vi "UI_(01)_Set_startup_controls_state.vi"(3 "error in (no error)":errorcluster, 4 "Settings cluster in":T1={"Defaults"={"Default User"=0.0, "VISA Resource Name "=""}, "Recording and saving"={"Researcher name"="", "Name prefix"="", "Data post-processing"={"Filter type"=enum."Savitzky-Golay", "Length"=31, "Order"=3}, "Stop at"=0.0, "\"Stop at\" enabled"=FALSE, "Default save folder path"=path "", "Acquisition FPS"=enum."Max"}, "Geometry"={"Cage diameter, mm"=0, "Starting angle MIDFIELD"=0, "Starting angle BORDER"=0, "Radius, mm CENTER"=0, "Radius, mm MIDFIELD"=0, "N segments MIDFIELD"=0, "N segments BORDER"=0, "R-gap, mm"=0.0, "Bridge swap"=FALSE, "Bridge H. offset"=0.0, "Bridge V. offset"=0.0, "Twisted neck"=FALSE, "Alt. magn. orientation"=FALSE, "Sensor board size"=enum."Small"}, "IO parameters"={"IO general config."=0, "IO 1 configuration"=0, "IO 2 configuration"=0, "IO 3 configuration"=0, "IO 4 configuration"=0, "Activate ext. RS-232"=0, "IO inversion config."=0, "Sync capability"=1}, "Conditions presets array"=[{"Enabled"=FALSE, "Name"="", "Specifier(s)"=[], "Response"={"Response type"=enum."Air puff", "TTL port"=enum."Port 1", "TTL pulse length, ms"=0.0}, "Has been set"=FALSE}, {"Enabled"=FALSE, "Name"="", "Specifier(s)"=[], "Response"={"Response type"=enum."Air puff", "TTL port"=enum."Port 1", "TTL pulse length, ms"=0.0}, "Has been set"=FALSE}, {"Enabled"=FALSE, "Name"="", "Specifier(s)"=[], "Response"={"Response type"=enum."Air puff", "TTL port"=enum."Port 1", "TTL pulse length, ms"=0.0}, "Has been set"=FALSE}, {"Enabled"=FALSE, "Name"="", "Specifier(s)"=[], "Response"={"Response type"=enum."Air puff", "TTL port"=enum."Port 1", "TTL pulse length, ms"=0.0}, "Has been set"=FALSE}, {"Enabled"=FALSE, "Name"="", "Specifier(s)"=[], "Response"={"Response type"=enum."Air puff", "TTL port"=enum."Port 1", "TTL pulse length, ms"=0.0}, "Has been set"=FALSE}, {"Enabled"=FALSE, "Name"="", "Specifier(s)"=[], "Response"={"Response type"=enum."Air puff", "TTL port"=enum."Port 1", "TTL pulse length, ms"=0.0}, "Has been set"=FALSE}, {"Enabled"=FALSE, "Name"="", "Specifier(s)"=[], "Response"={"Response type"=enum."Air puff", "TTL port"=enum."Port 1", "TTL pulse length, ms"=0.0}, "Has been set"=FALSE}, {"Enabled"=FALSE, "Name"="", "Specifier(s)"=[], "Response"={"Response type"=enum."Air puff", "TTL port"=enum."Port 1", "TTL pulse length, ms"=0.0}, "Has been set"=FALSE}, {"Enabled"=FALSE, "Name"="", "Specifier(s)"=[], "Response"={"Response type"=enum."Air puff", "TTL port"=enum."Port 1", "TTL pulse length, ms"=0.0}, "Has been set"=FALSE}, {"Enabled"=FALSE, "Name"="", "Specifier(s)"=[], "Response"={"Response type"=enum."Air puff", "TTL port"=enum."Port 1", "TTL pulse length, ms"=0.0}, "Has been set"=FALSE}, {"Enabled"=FALSE, "Name"="", "Specifier(s)"=[], "Response"={"Response type"=enum."Air puff", "TTL port"=enum."Port 1", "TTL pulse length, ms"=0.0}, "Has been set"=FALSE}, {"Enabled"=FALSE, "Name"="", "Specifier(s)"=[], "Response"={"Response type"=enum."Air puff", "TTL port"=enum."Port 1", "TTL pulse length, ms"=0.0}, "Has been set"=FALSE}, {"Enabled"=FALSE, "Name"="", "Specifier(s)"=[], "Response"={"Response type"=enum."Air puff", "TTL port"=enum."Port 1", "TTL pulse length, ms"=0.0}, "Has been set"=FALSE}, {"Enabled"=FALSE, "Name"="", "Specifier(s)"=[], "Response"={"Response type"=enum."Air puff", "TTL port"=enum."Port 1", "TTL pulse length, ms"=0.0}, "Has been set"=FALSE}], "Calibration parameters"={"Timing calibration sw/hw"=1.0, "True FPS"=80.0, "True frame time, s"=80.0, "Disp. calibration info"=[]}, "Settings loaded OK"=FALSE} {"Calibration parameters"."True frame time, s" format="%.10g"; "Calibration parameters"."Disp. calibration info"."Speed, µl per ms" format="%.3g"; "Calibration parameters"."True FPS" format="%.10g"; "Calibration parameters"."Timing calibration sw/hw" format="%.10g"; "Conditions presets array"."Specifier(s)"."Validity criteria(s)"."Validity value" min=0.0 step=0.1 format="%.2g"; "Conditions presets array"."Specifier(s)"."Value" step=1.0 format="%#.2g"; "Recording and saving"."Data post-processing"."Order" min=3 max=11 step=2; "Recording and saving"."Data post-processing"."Length" min=5 max=301 step=2; "Geometry"."Cage diameter, mm" scale=0.0..340.0}, 5 "All references in":T18) -> (0 "error out":errorcluster, 1 "Settings cluster out":T1={"Defaults"={"Default User"=0.0, "VISA Resource Name "=""}, "Recording and saving"={"Researcher name"="", "Name prefix"="", "Data post-processing"={"Filter type"=enum."Savitzky-Golay", "Length"=31, "Order"=3}, "Stop at"=0.0, "\"Stop at\" enabled"=FALSE, "Default save folder path"=path "", "Acquisition FPS"=enum."Max"}, "Geometry"={"Cage diameter, mm"=0, "Starting angle MIDFIELD"=0, "Starting angle BORDER"=0, "Radius, mm CENTER"=0, "Radius, mm MIDFIELD"=0, "N segments MIDFIELD"=0, "N segments BORDER"=0, "R-gap, mm"=0.0, "Bridge swap"=FALSE, "Bridge H. offset"=0.0, "Bridge V. offset"=0.0, "Twisted neck"=FALSE, "Alt. magn. orientation"=FALSE, "Sensor board size"=enum."Small"}, "IO parameters"={"IO general config."=0, "IO 1 configuration"=0, "IO 2 configuration"=0, "IO 3 configuration"=0, "IO 4 configuration"=0, "Activate ext. RS-232"=0, "IO inversion config."=0, "Sync capability"=1}, "Conditions presets array"=[{"Enabled"=FALSE, "Name"="", "Specifier(s)"=[], "Response"={"Response type"=enum."Air puff", "TTL port"=enum."Port 1", "TTL pulse length, ms"=0.0}, "Has been set"=FALSE}, {"Enabled"=FALSE, "Name"="", "Specifier(s)"=[], "Response"={"Response type"=enum."Air puff", "TTL port"=enum."Port 1", "TTL pulse length, ms"=0.0}, "Has been set"=FALSE}, {"Enabled"=FALSE, "Name"="", "Specifier(s)"=[], "Response"={"Response type"=enum."Air puff", "TTL port"=enum."Port 1", "TTL pulse length, ms"=0.0}, "Has been set"=FALSE}, {"Enabled"=FALSE, "Name"="", "Specifier(s)"=[], "Response"={"Response type"=enum."Air puff", "TTL port"=enum."Port 1", "TTL pulse length, ms"=0.0}, "Has been set"=FALSE}, {"Enabled"=FALSE, "Name"="", "Specifier(s)"=[], "Response"={"Response type"=enum."Air puff", "TTL port"=enum."Port 1", "TTL pulse length, ms"=0.0}, "Has been set"=FALSE}, {"Enabled"=FALSE, "Name"="", "Specifier(s)"=[], "Response"={"Response type"=enum."Air puff", "TTL port"=enum."Port 1", "TTL pulse length, ms"=0.0}, "Has been set"=FALSE}, {"Enabled"=FALSE, "Name"="", "Specifier(s)"=[], "Response"={"Response type"=enum."Air puff", "TTL port"=enum."Port 1", "TTL pulse length, ms"=0.0}, "Has been set"=FALSE}, {"Enabled"=FALSE, "Name"="", "Specifier(s)"=[], "Response"={"Response type"=enum."Air puff", "TTL port"=enum."Port 1", "TTL pulse length, ms"=0.0}, "Has been set"=FALSE}, {"Enabled"=FALSE, "Name"="", "Specifier(s)"=[], "Response"={"Response type"=enum."Air puff", "TTL port"=enum."Port 1", "TTL pulse length, ms"=0.0}, "Has been set"=FALSE}, {"Enabled"=FALSE, "Name"="", "Specifier(s)"=[], "Response"={"Response type"=enum."Air puff", "TTL port"=enum."Port 1", "TTL pulse length, ms"=0.0}, "Has been set"=FALSE}, {"Enabled"=FALSE, "Name"="", "Specifier(s)"=[], "Response"={"Response type"=enum."Air puff", "TTL port"=enum."Port 1", "TTL pulse length, ms"=0.0}, "Has been set"=FALSE}, {"Enabled"=FALSE, "Name"="", "Specifier(s)"=[], "Response"={"Response type"=enum."Air puff", "TTL port"=enum."Port 1", "TTL pulse length, ms"=0.0}, "Has been set"=FALSE}, {"Enabled"=FALSE, "Name"="", "Specifier(s)"=[], "Response"={"Response type"=enum."Air puff", "TTL port"=enum."Port 1", "TTL pulse length, ms"=0.0}, "Has been set"=FALSE}, {"Enabled"=FALSE, "Name"="", "Specifier(s)"=[], "Response"={"Response type"=enum."Air puff", "TTL port"=enum."Port 1", "TTL pulse length, ms"=0.0}, "Has been set"=FALSE}], "Calibration parameters"={"Timing calibration sw/hw"=1.0, "True FPS"=80.0, "True frame time, s"=80.0, "Disp. calibration info"=[]}, "Settings loaded OK"=FALSE} {"Calibration parameters"."True frame time, s" format="%.10g"; "Calibration parameters"."Disp. calibration info"."Speed, µl per ms" format="%.3g"; "Calibration parameters"."True FPS" format="%.10g"; "Calibration parameters"."Timing calibration sw/hw" format="%.10g"; "Conditions presets array"."Specifier(s)"."Validity criteria(s)"."Validity value" min=0.0 step=0.1 format="%.2g"; "Conditions presets array"."Specifier(s)"."Value" step=1.0 format="%#.2g"; "Recording and saving"."Data post-processing"."Order" min=3 max=11 step=2; "Recording and saving"."Data post-processing"."Length" min=5 max=301 step=2; "Geometry"."Cage diameter, mm" scale=0.0..340.0}, 2 "All references out":T18)   [LabVIEW 2018, in "Tracker.lvlib"]
uses:
  Tracker.lvlib
  Controls/CTL_All_References.ctl
  Controls/CTL_Controls_References.ctl
  Controls/CTL_Indicators_References.ctl
  Controls/CTL_Panes_and_VIs_References.ctl
  Controls/CTL_Histogram_Properties.ctl
  <vilib>/Utility/miscctls.llb/LVRangeTypeDef.ctl
  Controls/CTL_Settings_cluster.ctl
  Controls/CTL_Filter_selector.ctl
  Controls/CTL_Acquisition_speed_selector.ctl
  Controls/CTL_Segmented_plot_parameters.ctl
  Controls/CTL_IO_params_cluster.ctl
  Controls/CTL_Conditions_Array.ctl
  Controls/CTL_Conditions_Cluster.ctl
  Controls/CTL_Condition_type.ctl
  Controls/CTL_Comparison_type.ctl
  Controls/CTL_Validity_check_criteria.ctl
  Controls/CTL_Response_info.ctl
  Controls/CTL_Condition_response_type.ctl
  Controls/CTL_Reponse_port_info.ctl
  Controls/CTL_Calibration_parameters.ctl
  Controls/CTL_Dispenser_calibration_info.ctl
  <vilib>/Utility/miscctls.llb/LVPointTypeDef.ctl
  <vilib>/Utility/error.llb/Error Cluster From Error Code.vi
  <vilib>/ErrorRing/Error Ring.xnode
panel:
  in  "Histogram initialization cluster":T16={"X Scale.Range"={"Minimum"=0.0, "Maximum"=13.0, "Increment"=1.0, "Minor Increment"=1.0, "Start"=0.0}, "Caption.Text"="Zone preference (normalized)", "X Scale.Offset and Multiplier:Multiplier"=1.0, "X Scale.Offset and Multiplier:Offset"=0.0, "X Scale.Scale Fit"=2, "X Scale.Display Format:Precision"=0, "Y Scale.Mapping Mode"=0, "Zones preference empty initialized array"=[0, 0, 0, 0, 0, 0, 0, 0, 0, 0, 0, 0, 0, 0], "Plot.Fill/Point Color"=15790320}
  out "Panes references":T21
  out "Controls references params":string[][](array[string])
  out "Indicators references params":string[][](array[string])
  out "Indicators references":T20
  out "Controls references":T19
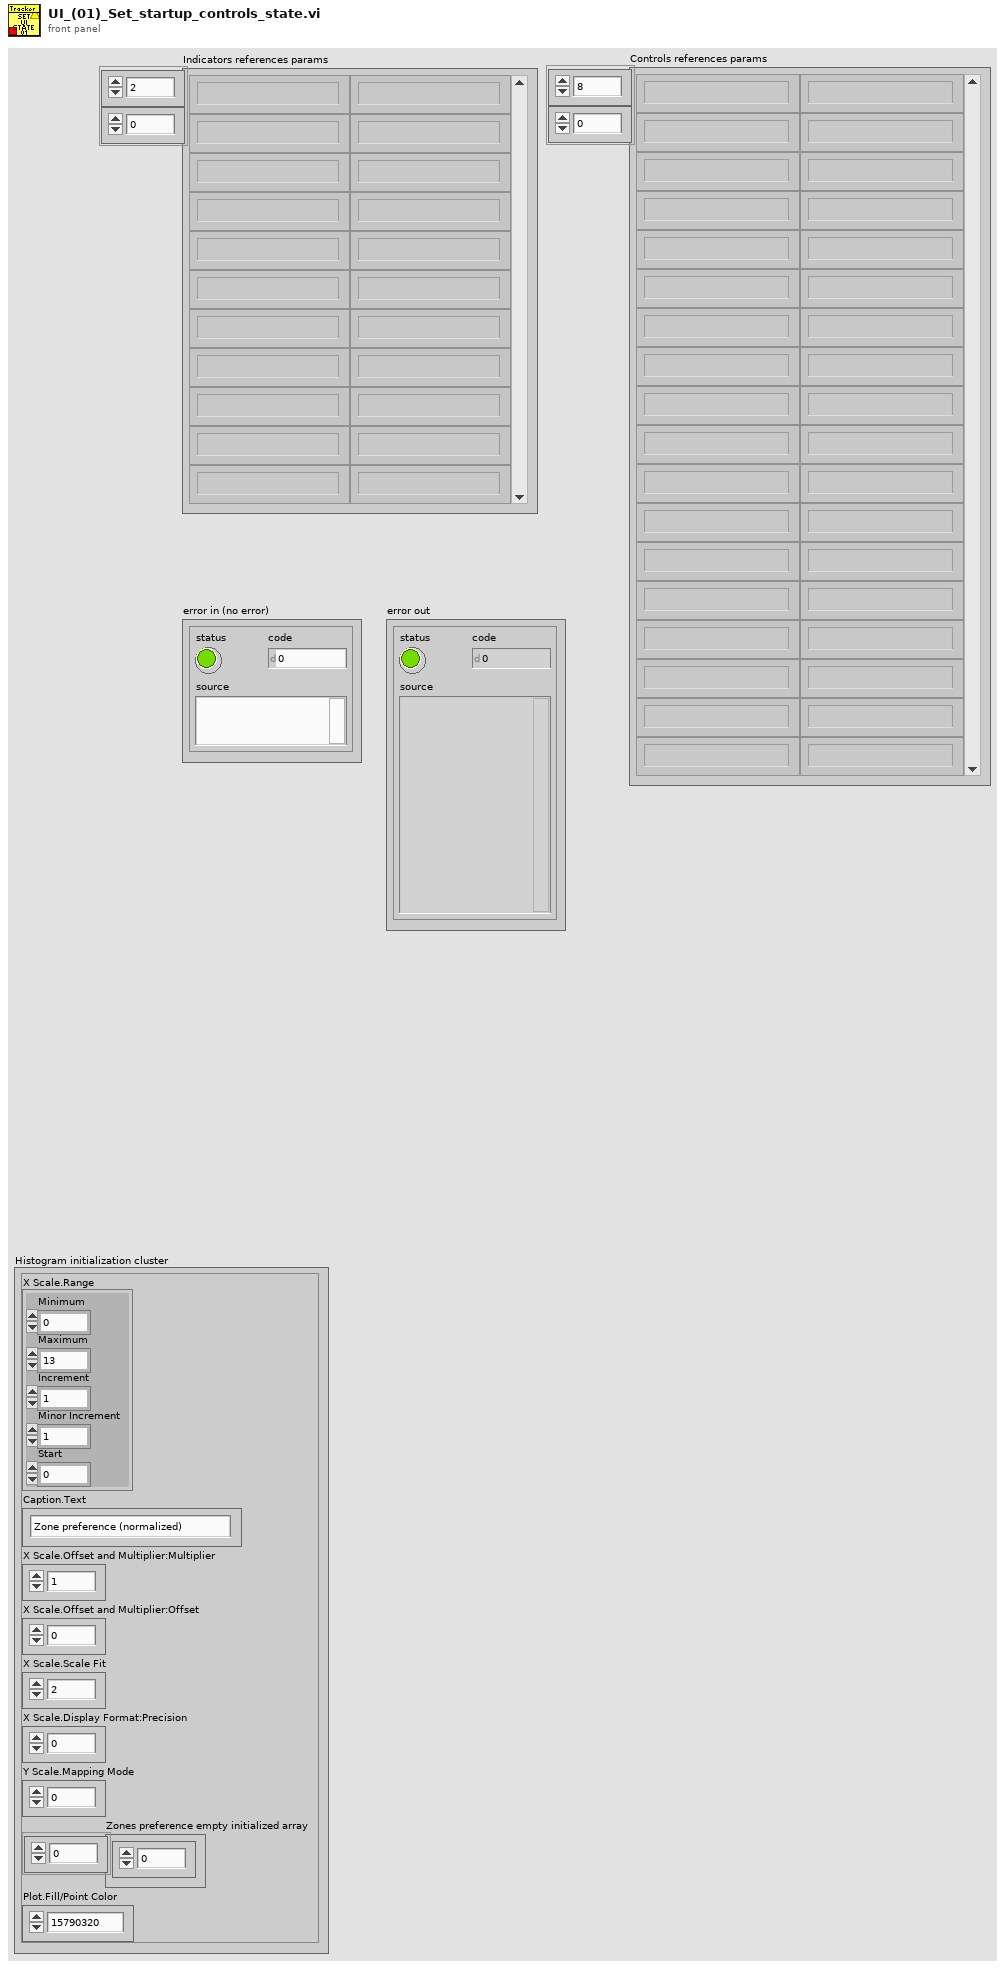
[diagram p1: front panel]
types:
  T1 = typedef "Tracker.lvlib/CTL_Settings_cluster.ctl" = cluster{"Defaults":cluster{"Default User":dbl, "VISA Resource Name ":string}, "Recording and saving":cluster{"Researcher name":string, "Name prefix":string, "Data post-processing":T2, "Stop at":dbl, "\"Stop at\" enabled":bool, "Default save folder path":path, "Acquisition FPS":T3}, "Geometry":T4, "IO parameters":T5, "Conditions presets array":T6, "Calibration parameters":T14, "Settings loaded OK":bool}
  T2 = typedef "Tracker.lvlib/CTL_Filter_selector.ctl" = cluster{"Filter type":enum16{"None", "Savitzky-Golay"}, "Length":i32, "Order":i32}
  T3 = typedef "Tracker.lvlib/CTL_Acquisition_speed_selector.ctl" = enum16{"Max", "Optimal", "Eco"}
  T4 = typedef "Tracker.lvlib/CTL_Segmented_plot_parameters.ctl" = cluster{"Cage diameter, mm":u16, "Starting angle MIDFIELD":i16, "Starting angle BORDER":i16, "Radius, mm CENTER":u16, "Radius, mm MIDFIELD":u16, "N segments MIDFIELD":u8, "N segments BORDER":u8, "R-gap, mm":sgl, "Bridge swap":bool, "Bridge H. offset":sgl, "Bridge V. offset":sgl, "Twisted neck":bool, "Alt. magn. orientation":bool, "Sensor board size":enum16{"Small", "Large"}}
  T5 = typedef "Tracker.lvlib/CTL_IO_params_cluster.ctl" = cluster{"IO general config.":u16, "IO 1 configuration":u16, "IO 2 configuration":u16, "IO 3 configuration":u16, "IO 4 configuration":u16, "Activate ext. RS-232":u16, "IO inversion config.":u16, "Sync capability":u8}
  T6 = typedef "Tracker.lvlib/CTL_Conditions_Array.ctl" = T7[]
  T7 = typedef "Tracker.lvlib/CTL_Conditions_Cluster.ctl" = cluster{"Enabled":bool, "Name":string, "Specifier(s)":cluster{"Specifier enabled":bool, "Condition type":T8, "Comparison type":T9, "Value":dbl, "Validity criteria(s)":cluster{"V. check enabled":bool, "Criteria":T10, "Validity value":dbl}[]}[], "Response":T11, "Has been set":bool}
  T8 = typedef "Tracker.lvlib/CTL_Condition_type.ctl" = enum16{"Speed", "Zone", "Angle to wall"}
  T9 = typedef "Tracker.lvlib/CTL_Comparison_type.ctl" = enum16{"Less", "Less or Equal", "Equal", "Greater or Equal", "Greater", "Not Equal"}
  T10 = typedef "Tracker.lvlib/CTL_Validity_check_criteria.ctl" = enum16{"Running bout (seconds)", "Running bout (meters)"}
  T11 = typedef "Tracker.lvlib/CTL_Response_info.ctl" = cluster{"Response type":T12, "TTL port":T13, "TTL pulse length, ms":dbl}
  T12 = typedef "Tracker.lvlib/CTL_Condition_response_type.ctl" = enum16{"None", "Air puff", "Liquid reward"}
  T13 = typedef "Tracker.lvlib/CTL_Reponse_port_info.ctl" = enum16{"Port 1", "Port 2", "Port 3", "Port 4"}
  T14 = typedef "Tracker.lvlib/CTL_Calibration_parameters.ctl" = cluster{"Timing calibration sw/hw":dbl, "True FPS":dbl, "True frame time, s":dbl, "Disp. calibration info":T15}
  T15 = typedef "Tracker.lvlib/CTL_Dispenser_calibration_info.ctl" = cluster{"Channel":u8, "Speed, µl per ms":dbl}[]
  T16 = typedef "Tracker.lvlib/CTL_Histogram_Properties.ctl" = cluster{"X Scale.Range":T17, "Caption.Text":string, "X Scale.Offset and Multiplier:Multiplier":dbl, "X Scale.Offset and Multiplier:Offset":dbl, "X Scale.Scale Fit":u8, "X Scale.Display Format:Precision":u8, "Y Scale.Mapping Mode":u8, "Zones preference empty initialized array":i32[], "Plot.Fill/Point Color":u32}
  T17 = typedef "LVRangeTypeDef.ctl" = cluster{"Minimum":dbl, "Maximum":dbl, "Increment":dbl, "Minor Increment":dbl, "Start":dbl}
  T18 = typedef "Tracker.lvlib/CTL_All_References.ctl" = cluster{"Controls references":T19, "Indicators references":T20, "Service references":T21}
  T19 = typedef "Tracker.lvlib/CTL_Controls_References.ctl" = cluster{"Check HW connection":refnum<vi>, "Save settings":refnum<vi>, "Reset zones":refnum<vi>, "Reset stimuli":refnum<vi>, "Record/Stop":refnum<vi>, "Reset barplot":refnum<vi>, "Multiplyer of chart RX":refnum<vi>, "Show zones":refnum<vi>, "Show magnets":refnum<vi>, "Show heatmap":refnum<vi>, "Show full track":refnum<vi>, "Open File":refnum<vi>, "Play/Pause":refnum<vi>, "Trace, s":refnum<vi>, "Playback speed":refnum<vi>, "Timeline":refnum<vi>, "By Zone stim. setup":refnum<vi>, "Set/Rec and Analyse Tab":refnum<vi>, "Cage radial segmentation":refnum<vi>, "Set IO config":refnum<vi>, "Rainbow (time)":refnum<vi>, "Rainbow (speed)":refnum<vi>, "Add Reward":refnum<vi>, "Modify Reward":refnum<vi>, "Delete Reward":refnum<vi>}
  T20 = typedef "Tracker.lvlib/CTL_Indicators_References.ctl" = cluster{"HW info":refnum<vi>, "Port":refnum<vi>, "Ready":refnum<vi>, "IO status indicator":refnum<vi>, "Current Time":refnum<vi>, "Record timestamp":refnum<vi>, "Mouse speed":refnum<vi>, "Mouse speed, mm/s":refnum<vi>, "Running, perc. of time":refnum<vi>, "Histograms":refnum<vi>, "Cage size":refnum<vi>, "Reward":refnum<vi>, "Current zone":refnum<vi>}
  T21 = typedef "Tracker.lvlib/CTL_Panes_and_VIs_References.ctl" = cluster{"Pane":refnum<vi>, "This VI":refnum<vi>, "Menu":refnum<k9>}
  T22 = typedef "LVPointTypeDef.ctl" = cluster{"Horizontal":i16, "Vertical":i16}
  T23 = enum8{"Enabled", "Disabled", "Disabled and Grayed Out"}
  T24 = enum32{"Page Enabled", "Page Disabled", "Page Disabled & Grayed"}
  T25 = cluster{"Slider":dbl, "Slider":dbl, "Slider":dbl}
  T26 = typedef "Tracker.lvlib/CTL_IO_status_indicator.ctl" = cluster{"IO1":bool, "IO2":bool, "IO3":bool, "IO4":bool, "St1":bool, "St2":bool, "St3":bool, "St4":bool, "Z1":bool, "Z2":bool, "Z3":bool, "Z4":bool, "Syn1":bool, "Syn2":bool, "RS-232 ext. activated":bool}
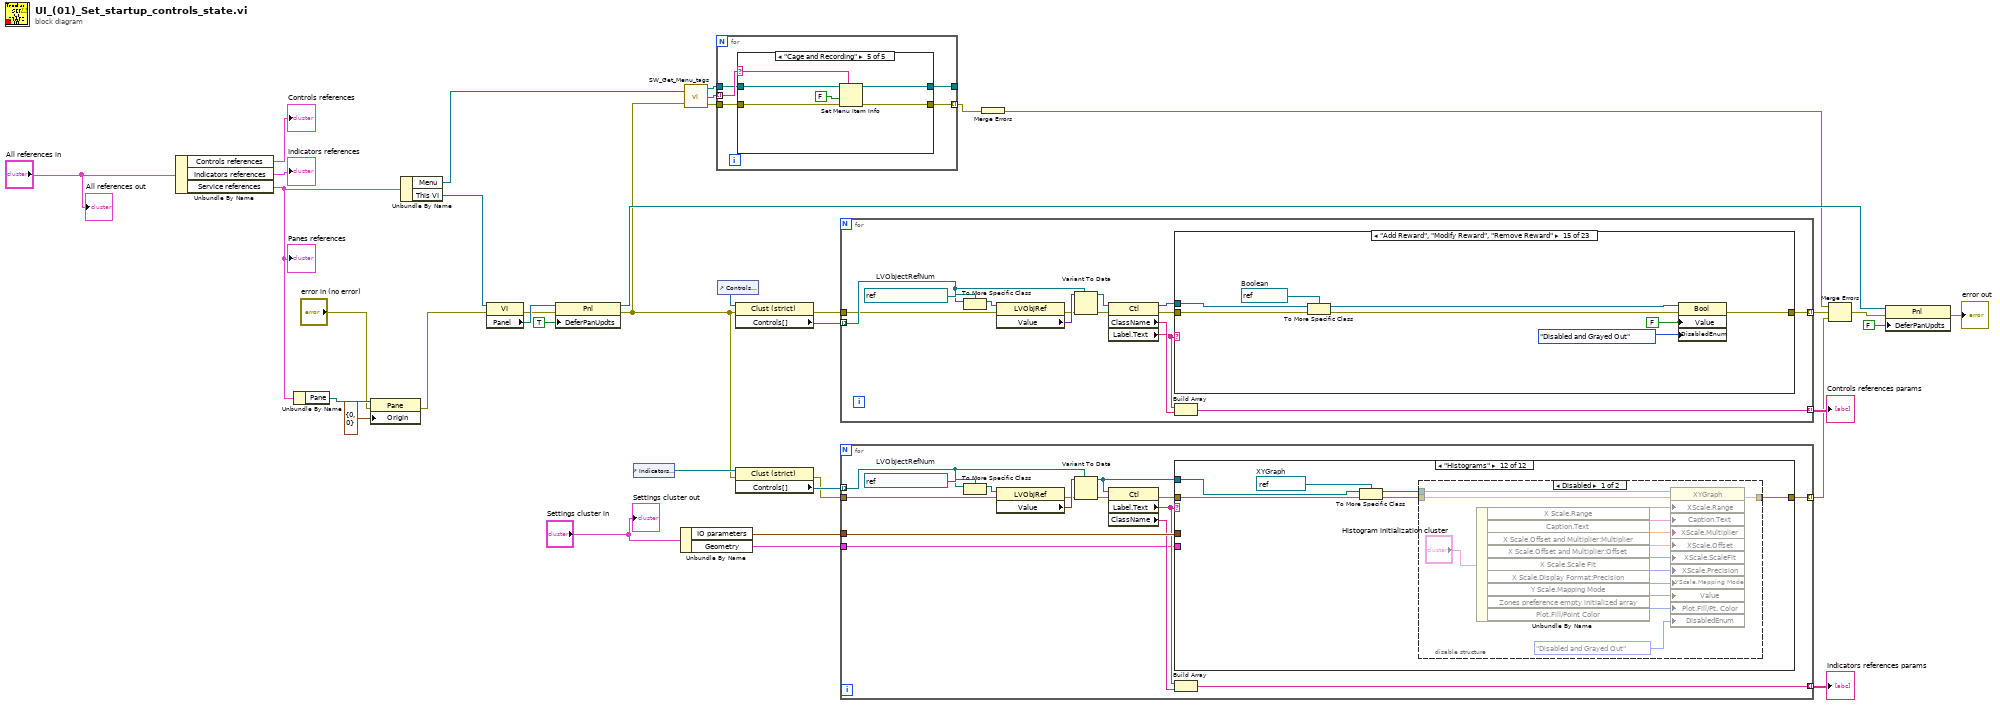
[diagram p0: block diagram]
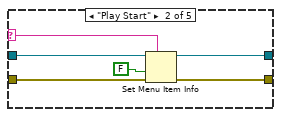
[diagram p3: hidden frame]
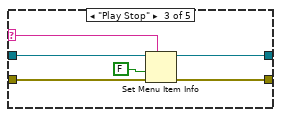
[diagram p4: hidden frame]
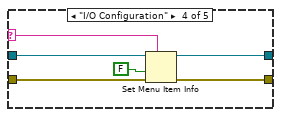
[diagram p5: hidden frame]
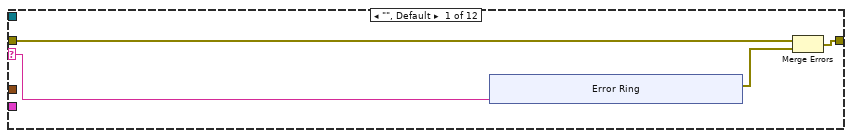
[diagram p6: hidden frame]
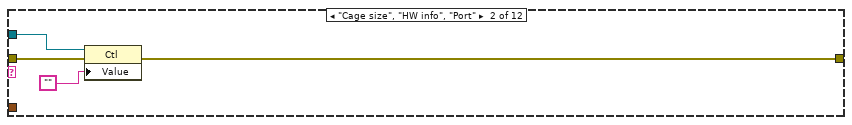
[diagram p7: hidden frame]
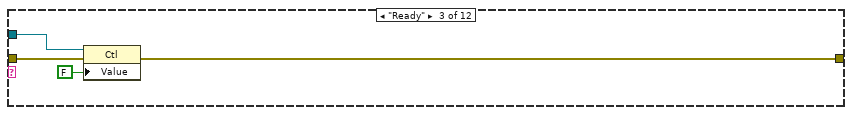
[diagram p8: hidden frame]
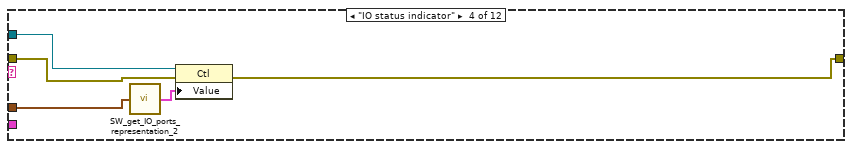
[diagram p9: hidden frame]
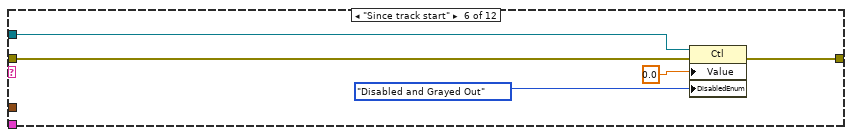
[diagram p11: hidden frame]
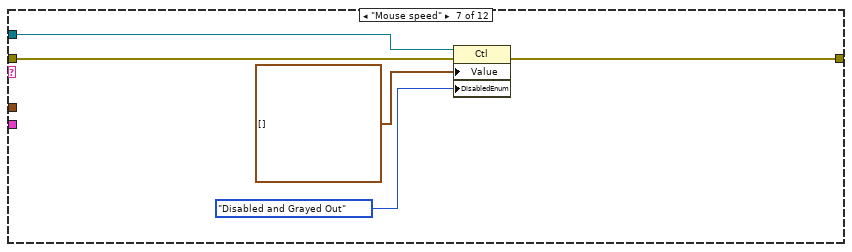
[diagram p12: hidden frame]
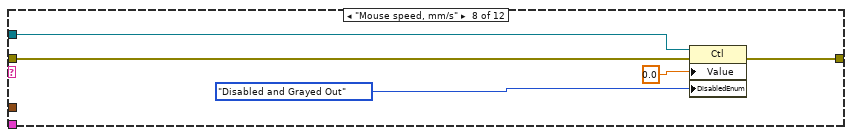
[diagram p13: hidden frame]
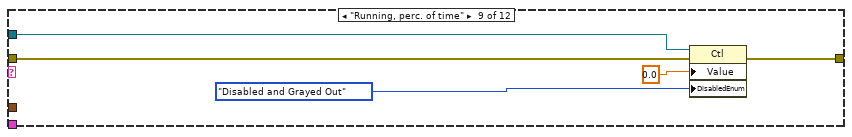
[diagram p14: hidden frame]
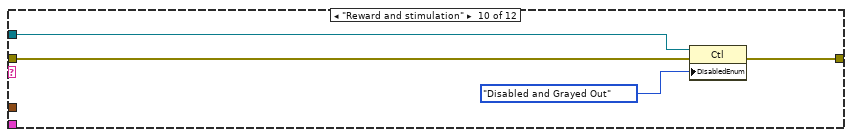
[diagram p15: hidden frame]
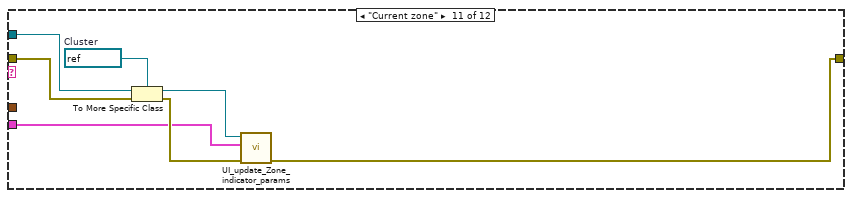
[diagram p16: hidden frame]
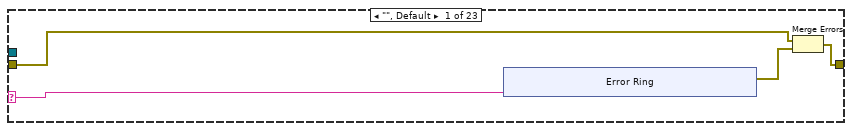
[diagram p18: hidden frame]
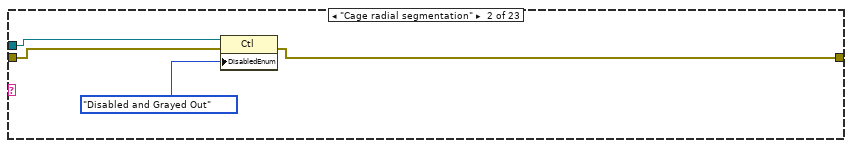
[diagram p19: hidden frame]
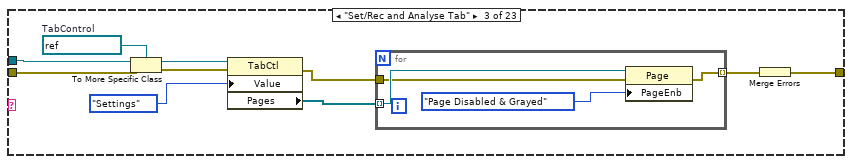
[diagram p20: hidden frame]
diagram:
  n1 = Unbundle By Name("All references in") -> ("Controls references"=→"Controls references":T19, "Indicators references"=→"Indicators references":T20, "Service references"=w14:T21)
  "Panes references" <- w14
  n2 = Unbundle By Name(w14) -> ("Pane"=w13:refnum<vi>)
  n3 = property class="Pane"(reference=w13, error in="error in (no error)", "Origin"=T22 {"Horizontal"=0, "Vertical"=0}) -> (error out=w11:errorcluster)  [unwired: 1 out]
  n4 = Unbundle By Name(w14) -> ("Menu"=w9:refnum<k9>, "This VI"=w25:refnum<vi>)
  n5 = property class="VI"(reference=w25, error in=w11) -> (error out=w18:errorcluster, "Panel"=w27:refnum<vi>)  [unwired: 1 out]
  n6 = property class="Pnl"(reference=w27, error in=w18, "DeferPanUpdts"=TRUE ("Defer Panel Updates")) -> (reference out=w19:refnum<vi>, error out=w8:errorcluster)
  n7 = control-ref of="Indicators references"() -> (w30:refnum<vi>)
  n8 = Unbundle By Name("Settings cluster in") -> ("IO parameters"=w15:T5, "Geometry"=w1:T4)
  n9 = call "SW_Get_Menu_tags.vi"("Menu ref in"=w9, "error in (no error)"=w8) -> ("Menu ref out"=w5:refnum<k9>, "(Sub)menu tags"=w7:string[], "error out"=w6:errorcluster)
  n10 = for {
    tunnel: w7 -> [w41] mode=indexing
    tunnel: w6 -> [w40]
    tunnel: [w39] -> w4 mode=indexing
    tunnel: [w38] -> _
    tunnel: w5 -> [w37]
    n11 = case shown="\"Cage and Recording\"" w41 {
      selector: w41 -> [_ w49 w55 w61 w67]
      tunnel: w40 -> [w43 w47 w53 w59 w65]
      tunnel: [w43 w46 w52 w58 w64] -> w39
      tunnel: [w42 w45 w51 w57 w63] -> w38
      tunnel: w37 -> [w42 w44 w50 w56 w62]
      frame "", Default {
      }
      frame "Play Start" {
        n12 = Set Menu Item Info(7:w49, 8:w47, 9:FALSE ("enabled"), 11:w44) -> (0:w46:errorcluster, 3:w45:refnum<k9>)  [unwired: 3 in]
      }
      frame "Play Stop" {
        n13 = Set Menu Item Info(7:w55, 8:w53, 9:FALSE ("enabled"), 11:w50) -> (0:w52:errorcluster, 3:w51:refnum<k9>)  [unwired: 3 in]
      }
      frame "I/O Configuration" {
        n14 = Set Menu Item Info(7:w61, 8:w59, 9:FALSE ("enabled"), 11:w56) -> (0:w58:errorcluster, 3:w57:refnum<k9>)  [unwired: 3 in]
      }
      frame "Cage and Recording" {
        n15 = Set Menu Item Info(7:w67, 8:w65, 9:FALSE ("enabled"), 11:w62) -> (0:w64:errorcluster, 3:w63:refnum<k9>)  [unwired: 3 in]
      }
    }
  }
  n16 = control-ref of="Controls references"() -> (w32:refnum<vi>)
  n17 = property class="Clust (strict)"(reference=w32, error in=w8) -> (error out=w24:errorcluster, "Controls[]"=w33:refnum<vi>[])  [unwired: 1 out]
  n18 = property class="Clust (strict)"(reference=w30, error in=w8) -> (error out=w23:errorcluster, "Controls[]"=w31:refnum<vi>[])  [unwired: 1 out]
  n19 = for {
    tunnel: w33 -> [w78] mode=indexing
    tunnel: [w75] -> w28 mode=indexing
    tunnel: w24 -> [w74]
    tunnel: [w70] -> w16 mode=indexing
    w80 = refnum<vi> refnum  # LVObjectRefNum
    n20 = To More Specific Class(target class=w80, reference=w78) -> (specific class reference=w81:refnum<vi>)  [unwired: 1 in, 1 out]
    n21 = property class="LVObjRef"(reference=w81, error in=w74) -> (error out=w73:errorcluster, "Value"=w79:variant)  [unwired: 1 out]
    n22 = Variant To Data(error in=w73, type=w78, Variant=w79) -> (data=w77:refnum<vi>, error out=w72:errorcluster)
    n23 = property class="Ctl"(reference=w77, error in=w72) -> (reference out=w68:refnum<vi>, error out=w69:errorcluster, "ClassName"=w76:string, "Label.Text"=w71:string)
    n24 = case shown="\"Add Reward\", \"Modify Reward\", \"Remove Reward\"" w71 {
      selector: w71 -> [w82 _ _ _ _ _ _ _ _ _ _ _ _ _ _ _ _ _ _ _ _ _ _]
      tunnel: [w84 w93 w97 w113 w121 w129 w137 w145 w153 w161 w169 w177 w185 w193 w201 w209 w217 w225 w233 w241 w249 w264 w271] -> w70
      tunnel: w69 -> [w85 w94 w101 w115 w123 w131 w139 w147 w155 w163 w171 w179 w187 w195 w203 w211 w219 w227 w235 w243 w251 w266 w273]
      tunnel: w68 -> [_ w96 w106 w118 w126 w134 w142 w150 w158 w166 w174 w182 w190 w198 w206 w214 w222 w230 w238 w246 w254 w269 w276]
      frame "", Default {
        n25 = xnode "Error Ring"("parameter 0"=w82) -> ("error out"=w83:errorcluster)
        n26 = Merge Errors(w85, w83) -> (w84:errorcluster)
      }
      frame "Cage radial segmentation" {
        n27 = property class="Ctl"(reference=w96, error in=w94, "DisabledEnum"=T23."Disabled and Grayed Out" ("Disabled")) -> (error out=w93:errorcluster)  [unwired: 1 out]
      }
      frame "Set/Rec and Analyse Tab" {
        w103 = refnum<vi> refnum  # TabControl
        n28 = To More Specific Class(target class=w103, reference=w106, error in=w101) -> (specific class reference=w104:refnum<vi>, error out=w100:errorcluster)
        n29 = property class="TabCtl"(reference=w104, error in=w100, "Value"=enum32{"Settings", "Recording and Analysis"}."Settings") -> (error out=w99:errorcluster, "Pages"=w102:refnum<vi>[])  [unwired: 1 out]
        n30 = for {
          tunnel: w102 -> [w109] mode=indexing
          tunnel: w99 -> [w108]
          tunnel: [w107] -> w98 mode=indexing
          n31 = property class="Page"(reference=w109, error in=w108, "PageEnb"=T24."Page Disabled & Grayed" ("Page Enabled State")) -> (error out=w107:errorcluster)  [unwired: 1 out]
        }
        n32 = Merge Errors(w98) -> (w97:errorcluster)
      }
      frame "Check HW connection" {
        w117 = refnum<vi> refnum  # Boolean
        n33 = To More Specific Class(target class=w117, reference=w118, error in=w115) -> (specific class reference=w116:refnum<vi>, error out=w114:errorcluster)
        n34 = property class="Bool"(reference=w116, error in=w114, "Value"=FALSE, "DisabledEnum"=T23."Disabled and Grayed Out" ("Disabled")) -> (error out=w113:errorcluster)  [unwired: 1 out]
      }
      frame "Save settings" {
        w125 = refnum<vi> refnum  # Boolean
        n35 = To More Specific Class(target class=w125, reference=w126, error in=w123) -> (specific class reference=w124:refnum<vi>, error out=w122:errorcluster)
        n36 = property class="Bool"(reference=w124, error in=w122, "Value"=FALSE, "DisabledEnum"=T23."Disabled and Grayed Out" ("Disabled")) -> (error out=w121:errorcluster)  [unwired: 1 out]
      }
      frame "Set IO config" {
        w133 = refnum<vi> refnum  # Boolean
        n37 = To More Specific Class(target class=w133, reference=w134, error in=w131) -> (specific class reference=w132:refnum<vi>, error out=w130:errorcluster)
        n38 = property class="Bool"(reference=w132, error in=w130, "Value"=FALSE, "DisabledEnum"=T23."Disabled and Grayed Out" ("Disabled")) -> (error out=w129:errorcluster)  [unwired: 1 out]
      }
      frame "Reset zones" {
        w141 = refnum<vi> refnum  # Boolean
        n39 = To More Specific Class(target class=w141, reference=w142, error in=w139) -> (specific class reference=w140:refnum<vi>, error out=w138:errorcluster)
        n40 = property class="Bool"(reference=w140, error in=w138, "Value"=FALSE, "DisabledEnum"=T23."Disabled and Grayed Out" ("Disabled")) -> (error out=w137:errorcluster)  [unwired: 1 out]
      }
      frame "Reset stimuli" {
        w149 = refnum<vi> refnum  # Boolean
        n41 = To More Specific Class(target class=w149, reference=w150, error in=w147) -> (specific class reference=w148:refnum<vi>, error out=w146:errorcluster)
        n42 = property class="Bool"(reference=w148, error in=w146, "Value"=FALSE, "DisabledEnum"=T23."Disabled and Grayed Out" ("Disabled")) -> (error out=w145:errorcluster)  [unwired: 1 out]
      }
      frame "Record/Stop" {
        w157 = refnum<vi> refnum  # Boolean
        n43 = To More Specific Class(target class=w157, reference=w158, error in=w155) -> (specific class reference=w156:refnum<vi>, error out=w154:errorcluster)
        n44 = property class="Bool"(reference=w156, error in=w154, "Value"=FALSE, "DisabledEnum"=T23."Disabled and Grayed Out" ("Disabled")) -> (error out=w153:errorcluster)  [unwired: 1 out]
      }
      frame "Reset barplot" {
        w165 = refnum<vi> refnum  # Boolean
        n45 = To More Specific Class(target class=w165, reference=w166, error in=w163) -> (specific class reference=w164:refnum<vi>, error out=w162:errorcluster)
        n46 = property class="Bool"(reference=w164, error in=w162, "Value"=FALSE, "DisabledEnum"=T23."Disabled and Grayed Out" ("Disabled")) -> (error out=w161:errorcluster)  [unwired: 1 out]
      }
      frame "Multiplyer of chart RX" {
        w173 = refnum<vi> refnum  # Slide
        n47 = To More Specific Class(target class=w173, reference=w174, error in=w171) -> (specific class reference=w172:refnum<vi>, error out=w170:errorcluster)
        n48 = property class="Slide"(reference=w172, error in=w170, "Value"=u8 1, "DisabledEnum"=T23."Disabled and Grayed Out" ("Disabled")) -> (error out=w169:errorcluster)  [unwired: 1 out]
      }
      frame "Show zones" {
        w181 = refnum<vi> refnum  # Boolean
        n49 = To More Specific Class(target class=w181, reference=w182, error in=w179) -> (specific class reference=w180:refnum<vi>, error out=w178:errorcluster)
        n50 = property class="Bool"(reference=w180, error in=w178, "Value"=TRUE, "DisabledEnum"=T23."Disabled and Grayed Out" ("Disabled")) -> (error out=w177:errorcluster)  [unwired: 1 out]
      }
      frame "Show magnets" {
        w189 = refnum<vi> refnum  # Boolean
        n51 = To More Specific Class(target class=w189, reference=w190, error in=w187) -> (specific class reference=w188:refnum<vi>, error out=w186:errorcluster)
        n52 = property class="Bool"(reference=w188, error in=w186, "Value"=TRUE, "DisabledEnum"=T23."Disabled and Grayed Out" ("Disabled")) -> (error out=w185:errorcluster)  [unwired: 1 out]
      }
      frame "Rainbow (speed)", "Rainbow (time)" {
        w197 = refnum<vi> refnum  # Boolean
        n53 = To More Specific Class(target class=w197, reference=w198, error in=w195) -> (specific class reference=w196:refnum<vi>, error out=w194:errorcluster)
        n54 = property class="Bool"(reference=w196, error in=w194, "Value"=FALSE, "DisabledEnum"=T23."Disabled and Grayed Out" ("Disabled")) -> (error out=w193:errorcluster)  [unwired: 1 out]
      }
      frame "Add Reward", "Modify Reward", "Remove Reward" {
        w205 = refnum<vi> refnum  # Boolean
        n55 = To More Specific Class(target class=w205, reference=w206, error in=w203) -> (specific class reference=w204:refnum<vi>, error out=w202:errorcluster)
        n56 = property class="Bool"(reference=w204, error in=w202, "Value"=FALSE, "DisabledEnum"=T23."Disabled and Grayed Out" ("Disabled")) -> (error out=w201:errorcluster)  [unwired: 1 out]
      }
      frame "Show heatmap" {
        w213 = refnum<vi> refnum  # Boolean
        n57 = To More Specific Class(target class=w213, reference=w214, error in=w211) -> (specific class reference=w212:refnum<vi>, error out=w210:errorcluster)
        n58 = property class="Bool"(reference=w212, error in=w210, "Value"=FALSE, "DisabledEnum"=T23."Disabled and Grayed Out" ("Disabled")) -> (error out=w209:errorcluster)  [unwired: 1 out]
      }
      frame "Show full track" {
        w221 = refnum<vi> refnum  # Boolean
        n59 = To More Specific Class(target class=w221, reference=w222, error in=w219) -> (specific class reference=w220:refnum<vi>, error out=w218:errorcluster)
        n60 = property class="Bool"(reference=w220, error in=w218, "Value"=FALSE, "DisabledEnum"=T23."Disabled and Grayed Out" ("Disabled")) -> (error out=w217:errorcluster)  [unwired: 1 out]
      }
      frame "Open File" {
        w229 = refnum<vi> refnum  # Boolean
        n61 = To More Specific Class(target class=w229, reference=w230, error in=w227) -> (specific class reference=w228:refnum<vi>, error out=w226:errorcluster)
        n62 = property class="Bool"(reference=w228, error in=w226, "Value"=FALSE, "DisabledEnum"=T23."Disabled and Grayed Out" ("Disabled")) -> (error out=w225:errorcluster)  [unwired: 1 out]
      }
      frame "Play/Pause" {
        w237 = refnum<vi> refnum  # Boolean
        n63 = To More Specific Class(target class=w237, reference=w238, error in=w235) -> (specific class reference=w236:refnum<vi>, error out=w234:errorcluster)
        n64 = property class="Bool"(reference=w236, error in=w234, "Value"=FALSE, "DisabledEnum"=T23."Disabled and Grayed Out" ("Disabled")) -> (error out=w233:errorcluster)  [unwired: 1 out]
      }
      frame "Trace, s" {
        w245 = refnum<vi> refnum  # Slide
        n65 = To More Specific Class(target class=w245, reference=w246, error in=w243) -> (specific class reference=w244:refnum<vi>, error out=w242:errorcluster)
        n66 = property class="Slide"(reference=w244, error in=w242, "Value"=u8 5, "DisabledEnum"=T23."Disabled and Grayed Out" ("Disabled")) -> (error out=w241:errorcluster)  [unwired: 1 out]
      }
      frame "Playback speed" {
        w253 = refnum<vi> refnum  # Ring
        n67 = To More Specific Class(target class=w253, reference=w254, error in=w251) -> (specific class reference=w252:refnum<vi>, error out=w250:errorcluster)
        n68 = property class="Ring"(reference=w252, error in=w250, "Value"=u8 3, "DisabledEnum"=T23."Disabled and Grayed Out" ("Disabled")) -> (error out=w249:errorcluster)  [unwired: 1 out]
      }
      frame "Timeline" {
        w255 = 0.0 ("Slider")
        w268 = refnum<vi> refnum  # Slide
        n69 = To More Specific Class(target class=w268, reference=w269, error in=w266) -> (specific class reference=w267:refnum<vi>, error out=w265:errorcluster)
        n70 = Bundle(cluster=T25 {"Slider"=0.0, "Slider"=0.0, "Slider"=0.0} ("Timeline"), "Slider"=w255, "Slider"=0.001, "Slider"=w255) -> (w261:T25)
        n71 = To Variant(anything=w261) -> (Variant=w260:variant)
        n72 = property class="Slide"(reference=w267, error in=w265, "Value"=w260, "DisabledEnum"=T23."Disabled and Grayed Out" ("Disabled"), "Scale.Minimum"=0.0 ("Scale.Range:Minimum"), "Scale.Maximum"=60.0 ("Scale.Range:Maximum"), "Scale.RngStart"=0.0 ("Scale.Range:Start")) -> (error out=w264:errorcluster)  [unwired: 1 out]
      }
      frame "By Zone stim. setup" {
        w275 = refnum<vi> refnum  # RadioButtonsControl
        n73 = To More Specific Class(target class=w275, reference=w276, error in=w273) -> (specific class reference=w274:refnum<vi>, error out=w272:errorcluster)
        n74 = property class="RadioBtnsControl"(reference=w274, error in=w272, "DisabledEnum"=T23."Disabled and Grayed Out" ("Disabled")) -> (error out=w271:errorcluster)  [unwired: 1 out]
      }
    }
    n75 = Build Array(w71, w76) -> (w75:string[])
  }
  "Controls references params" <- w28
  n76 = for {
    tunnel: w31 -> [w288] mode=indexing
    tunnel: [w278] -> w29 mode=indexing
    tunnel: w23 -> [w286]
    tunnel: [w282] -> w22 mode=indexing
    tunnel: w15 -> [w281]
    tunnel: w1 -> [w277]
    w290 = refnum<vi> refnum  # LVObjectRefNum
    n77 = To More Specific Class(target class=w290, reference=w288) -> (specific class reference=w291:refnum<vi>)  [unwired: 1 in, 1 out]
    n78 = property class="LVObjRef"(reference=w291, error in=w286) -> (error out=w285:errorcluster, "Value"=w289:variant)  [unwired: 1 out]
    n79 = Variant To Data(error in=w285, type=w288, Variant=w289) -> (data=w287:refnum<vi>, error out=w284:errorcluster)
    n80 = property class="Ctl"(reference=w287, error in=w284) -> (error out=w283:errorcluster, "Label.Text"=w280:string, "ClassName"=w279:string)  [unwired: 1 out]
    n81 = case shown="\"Histograms\"" w280 {
      selector: w280 -> [w292 _ _ _ _ _ _ _ _ _ _ _]
      tunnel: w287 -> [_ w306 w310 w312 _ w321 w326 w331 w336 w340 w345 w353]
      tunnel: w283 -> [w295 w305 w309 w313 w316 w320 w325 w330 w335 w339 w344 w349]
      tunnel: [w294 w304 w308 w315 w316 w319 w324 w329 w334 w338 w347 w352] -> w282
      tunnel: w281 -> [_ _ _ w314 _ _ _ _ _ _ _ _]
      tunnel: w277 -> [_ _ _ _ _ _ _ _ _ _ w341 _]
      frame "", Default {
        n82 = xnode "Error Ring"("parameter 0"=w292) -> ("error out"=w293:errorcluster)
        n83 = Merge Errors(w295, w293) -> (w294:errorcluster)
      }
      frame "Cage size", "HW info", "Port" {
        n84 = property class="Ctl"(reference=w306, error in=w305, "Value"="") -> (error out=w304:errorcluster)  [unwired: 1 out]
      }
      frame "Ready" {
        n85 = property class="Ctl"(reference=w310, error in=w309, "Value"=FALSE) -> (error out=w308:errorcluster)  [unwired: 1 out]
      }
      frame "IO status indicator" {
        n86 = call "SW_get_IO_ports_representation_2.vi"("Sync parameters cluster input"=w314) -> ("IO status indicator"=w311:T26)
        n87 = property class="Ctl"(reference=w312, error in=w313, "Value"=w311) -> (error out=w315:errorcluster)  [unwired: 1 out]
      }
      frame "Current Time" {
      }
      frame "Since track start" {
        n88 = property class="Ctl"(reference=w321, error in=w320, "Value"=0.0, "DisabledEnum"=T23."Disabled and Grayed Out" ("Disabled")) -> (error out=w319:errorcluster)  [unwired: 1 out]
      }
      frame "Mouse speed" {
        n89 = property class="Ctl"(reference=w326, error in=w325, "Value"=waveform(dbl)[] [] ("History Data"), "DisabledEnum"=T23."Disabled and Grayed Out" ("Disabled")) -> (error out=w324:errorcluster)  [unwired: 1 out]
      }
      frame "Mouse speed, mm/s" {
        n90 = property class="Ctl"(reference=w331, error in=w330, "Value"=0.0, "DisabledEnum"=T23."Disabled and Grayed Out" ("Disabled")) -> (error out=w329:errorcluster)  [unwired: 1 out]
      }
      frame "Running, perc. of time" {
        n91 = property class="Ctl"(reference=w336, error in=w335, "Value"=0.0, "DisabledEnum"=T23."Disabled and Grayed Out" ("Disabled")) -> (error out=w334:errorcluster)  [unwired: 1 out]
      }
      frame "Reward and stimulation" {
        n92 = property class="Ctl"(reference=w340, error in=w339, "DisabledEnum"=T23."Disabled and Grayed Out" ("Disabled")) -> (error out=w338:errorcluster)  [unwired: 1 out]
      }
      frame "Current zone" {
        w346 = refnum<vi> refnum  # Cluster
        n93 = To More Specific Class(target class=w346, reference=w345, error in=w344) -> (specific class reference=w342:refnum<vi>, error out=w343:errorcluster)
        n94 = call "UI_update_Zone_indicator_params.vi"("error in (no error)"=w343, "Geometry params in"=w341, "Zone indicator ref. in"=w342) -> ("error out"=w347:errorcluster)  [unwired: 7 in, 1 out]
      }
      frame "Histograms" {
        w350 = refnum<vi> refnum  # XYGraph
        n95 = To More Specific Class(target class=w350, reference=w353, error in=w349) -> (specific class reference=w351:refnum<vi>, error out=w348:errorcluster)
        n96 = disable-structure shown="Disabled" {
          disable-tunnel: [w367 _] -> w352
          disable-tunnel: w351 -> [w366 _]
          disable-tunnel: w348 -> [w355 _]
          frame Disabled {
            n97 = Unbundle By Name("Histogram initialization cluster") -> ("X Scale.Range"=w364:T17, "Caption.Text"=w363:string, "X Scale.Offset and Multiplier:Multiplier"=w362:dbl, "X Scale.Offset and Multiplier:Offset"=w361:dbl, "X Scale.Scale Fit"=w360:u8, "X Scale.Display Format:Precision"=w359:u8, "Y Scale.Mapping Mode"=w358:u8, "Zones preference empty initialized array"=w357:i32[], "Plot.Fill/Point Color"=w356:u32)
            n98 = property class="XYGraph"(reference=w366, error in=w355, "XScale.Range"=w364, "Caption.Text"=w363, "XScale.Multiplier"=w362, "XScale.Offset"=w361, "XScale.ScaleFit"=w360, "XScale.Precision"=w359, "YScale.Mapping Mode"=w358, "Value"=w357, "Plot.Fill/Pt. Color"=w356, "DisabledEnum"=T23."Disabled and Grayed Out" ("Disabled")) -> (error out=w367:errorcluster)  [unwired: 1 out]
          }
          frame Enabled {
          }
        }
      }
    }
    n99 = Build Array(w280, w279) -> (w278:string[])
  }
  "Indicators references params" <- w29
  n100 = Merge Errors(w4) -> (w3:errorcluster)
  n101 = Merge Errors(w3, w16, w22) -> (w21:errorcluster)
  n102 = property class="Pnl"(reference=w19, error in=w21, "DeferPanUpdts"=FALSE ("Defer Panel Updates")) -> (error out=→"error out":errorcluster)  [unwired: 1 out]
  "All references out" <- "All references in"
  "Settings cluster out" <- "Settings cluster in"
